vi "LoadImages.vi"(6 "usb":bool, 8 "Background Img":T1, 9 "Background Path":path, 10 "Reference Img":T1, 11 "Reference Path":path) -> ()   [LabVIEW 2013]
uses:
  <vilib>/vision/Image Controls.llb/IMAQ Image.ctl
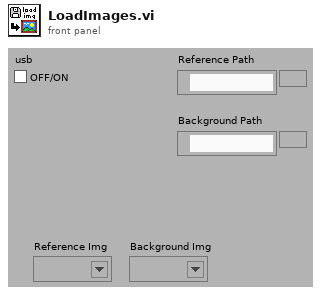
[diagram p1: front panel]
types:
  T1 = typedef "IMAQ Image.ctl" = refnum<image>
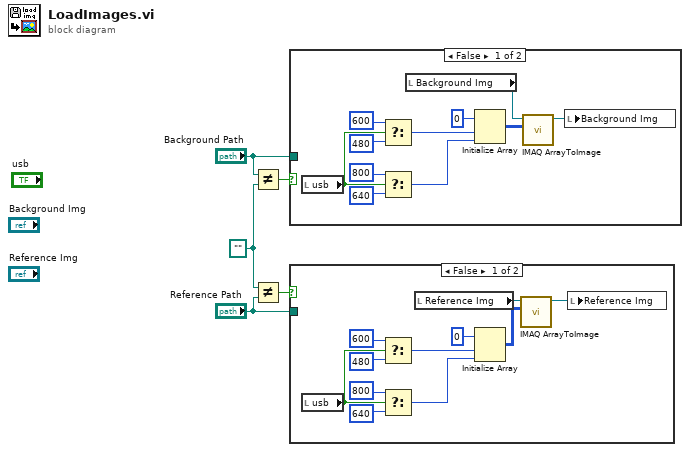
[diagram p0: block diagram]
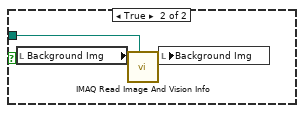
[diagram p2: hidden frame]
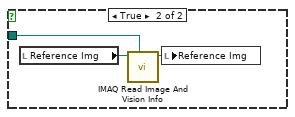
[diagram p3: hidden frame]
diagram:
  w3 = path ""
  n1 = Not Equal?(x="Background Path", y=w3) -> (x != y?=w4:bool)
  n2 = Not Equal?(x=w3, y="Reference Path") -> (x != y?=w5:bool)
  n3 = case shown="False" w4 {
    tunnel: "Background Path" -> [_ w19]
    frame False {
      n4 = local read "usb"() -> (w8:bool)
      n5 = Select(t=600 ("dimension size"), s=w8, f=480 ("dimension size")) -> (s? t:f=w7:i32)
      n6 = Select(t=800 ("dimension size"), s=w8, f=640 ("dimension size")) -> (s? t:f=w6:i32)
      n7 = local read "Background Img"() -> (w13:T1)
      n8 = Initialize Array(u8 0 ("element"), w7, w6) -> (w15:u8[][])
      n9 = call "IMAQ ArrayToImage"("Image Pixels (U8)"=w15, "Image"=w13) -> ("Image Out"=w16:T1)  [unwired: 8 in, 1 out]
      n10 = local write "Background Img"(w16) -> ()
    }
    frame True {
      n11 = local read "Background Img"() -> (w17:T1)
      n12 = call "IMAQ Read Image And Vision Info"("File Path"=w19, "Image"=w17) -> ("Image Out"=w18:T1)  [unwired: 7 in, 2 out]
      n13 = local write "Background Img"(w18) -> ()
    }
  }
  n14 = case shown="False" w5 {
    tunnel: "Reference Path" -> [_ w33]
    frame False {
      n15 = local read "usb"() -> (w26:bool)
      n16 = Select(t=600 ("dimension size"), s=w26, f=480 ("dimension size")) -> (s? t:f=w21:i32)
      n17 = Select(t=800 ("dimension size"), s=w26, f=640 ("dimension size")) -> (s? t:f=w20:i32)
      n18 = local read "Reference Img"() -> (w27:T1)
      n19 = Initialize Array(u8 0 ("element"), w21, w20) -> (w29:u8[][])
      n20 = call "IMAQ ArrayToImage"("Image Pixels (U8)"=w29, "Image"=w27) -> ("Image Out"=w28:T1)  [unwired: 8 in, 1 out]
      n21 = local write "Reference Img"(w28) -> ()
    }
    frame True {
      n22 = local read "Reference Img"() -> (w31:T1)
      n23 = call "IMAQ Read Image And Vision Info"("File Path"=w33, "Image"=w31) -> ("Image Out"=w32:T1)  [unwired: 7 in, 2 out]
      n24 = local write "Reference Img"(w32) -> ()
    }
  }
